vi "HandleGroundPass.vi"(7 "InitState":T1=enum."Pass", 8 "error in":errorcluster, 11 "Toggle?":bool) -> (0 "error out":errorcluster, 3 "State":T1=enum."Pass")   [LabVIEW 2015]
uses:
  PassState.ctl
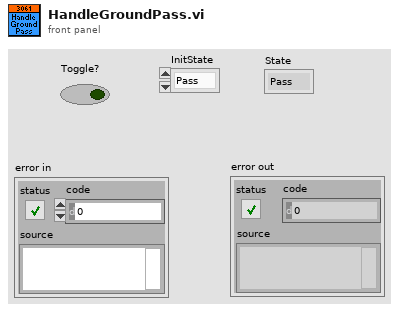
[diagram p1: front panel]
types:
  T1 = typedef "PassState.ctl" = enum16{"Stop", "Pass"}
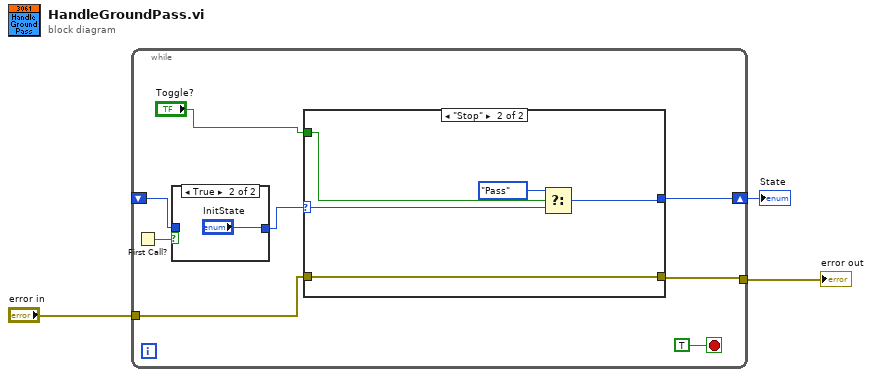
[diagram p0: block diagram]
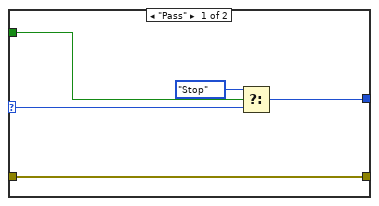
[diagram p3: hidden frame]
diagram:
  n1 = while {
    tunnel: "error in" -> [w9]
    tunnel: [w8] -> w2
    shift-right: [w6] -> w1
    shift-left: _ -> [w5]
    stop <- TRUE stop-if-true
    n2 = First Call?() -> (First Call?: T/F=w10:bool)
    n3 = case shown="True" w10 {
      tunnel: w5 -> [w12 _]
      tunnel: [w12 "InitState"] -> w7
      frame False {
      }
      frame True {
      }
    }
    n4 = case shown="\"Stop\"" w7 {
      selector: w7 -> [w15 w23]
      tunnel: w9 -> [w17 w20]
      tunnel: [w17 w20] -> w8
      tunnel: [w18 w21] -> w6
      tunnel: "Toggle?" -> [w16 w22]
      frame "Pass" {
        n5 = Select(t=PassState."Stop", s=w16, f=w15) -> (s? t:f=w18:T1)
      }
      frame "Stop" {
        n6 = Select(t=PassState."Pass", s=w22, f=w23) -> (s? t:f=w21:T1)
      }
    }
  }
  "error out" <- w2
  "State" <- w1
